vi "sv_Buffer Even-Angle Signal (N Ch).vi"(0 "initial buffered x[n]":dbl[][](array[numeric]), 1 "reset? (True)":bool=TRUE, 5 "even-angle signals":cluster{"r0":dbl, "dr":dbl, "Y":dbl[]}[](array[cluster]) {"r0" format="%.2p"; "dr" format="%.2p"; "Y" format="%.2f"}, 9 "integration cycles":u32) -> (3 "buffered x[n]":dbl[][](array[numeric]), 4 "buffered x[n] for analysis":dbl[][](array[numeric]), 6 "sample rate":dbl)   [LabVIEW 2017]
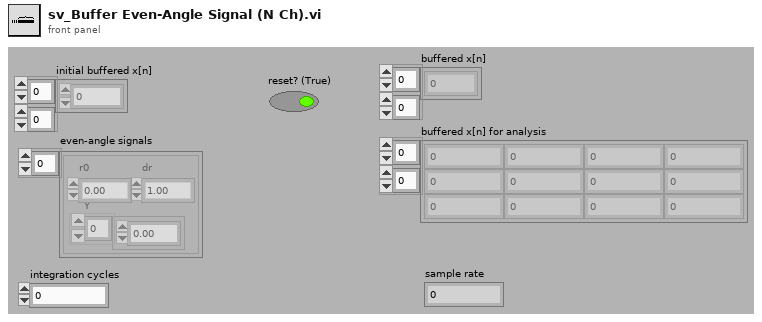
[diagram p1: front panel]
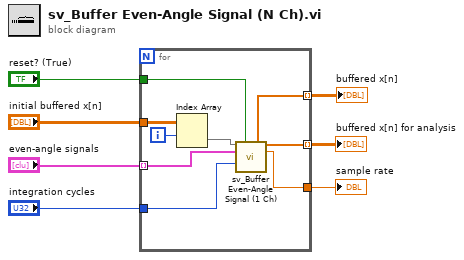
[diagram p0: block diagram]
diagram:
  n1 = for {
    tunnel: "even-angle signals" -> [w10] mode=indexing
    tunnel: "initial buffered x[n]" -> [w12]
    tunnel: "integration cycles" -> [w16]
    tunnel: "reset? (True)" -> [w15]
    tunnel: [w14] -> w3 mode=indexing
    tunnel: [w13] -> w2
    tunnel: [w8] -> w1 mode=indexing
    i -> [w11]
    n2 = Index Array(array=w12, index (row)=w11) -> (element=w9:dbl[])  [unwired: 1 in]
    n3 = call <vilib>:"sv_Buffer Even-Angle Signal (1 Ch).vi"("initial buffered x[n]"=w9, "reset? (True)"=w15, "even-angle signal"=w10, "integration cycles"=w16) -> ("buffered x[n]"=w8:dbl[], "buffered x[n] for analysis"=w14:dbl[], "sample rate"=w13:dbl)  [unwired: 9 in]
  }
  "buffered x[n] for analysis" <- w3
  "sample rate" <- w2
  "buffered x[n]" <- w1
